vi "4155C Config Chart Colours.vi"(4 "Numeric":i32, 7 "XY Graph 2":refnum<vi>) -> ()   [LabVIEW 2019]
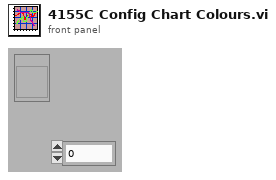
[diagram p1: front panel]
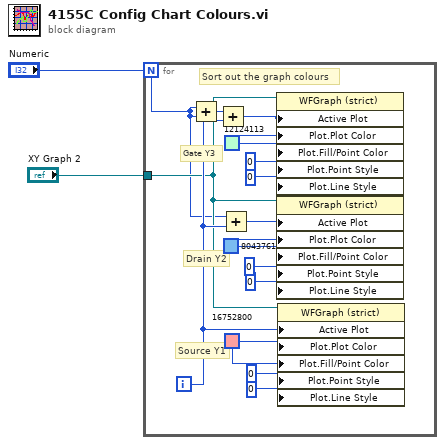
[diagram p0: block diagram]
diagram:
  n1 = for {
    N: "Numeric" -> [w3]
    tunnel: "XY Graph 2" -> [w6]
    i -> [w16]
    w15 = u32 16752800
    w14 = u32 8043761
    w13 = u32 12124113
    # "Sort out the graph colours"
    # "Source Y1"
    # "Drain Y2"
    # "Gate Y3"
    n2 = Add(x=w3, y=w3) -> (x+y=w17:i32)
    n3 = Add(x=w17, y=w16) -> (x+y=w5:i32)
    n4 = Add(x=w3, y=w16) -> (x+y=w4:i32)
    n5 = property on="Property Node" class="WFGraph (strict)"(reference=w6, "Active Plot"=w5, "Plot.Plot Color"=w13, "Plot.Fill/Point Color"=w13, "Plot.Point Style"=u8 0, "Plot.Line Style"=u8 0) -> ()  [unwired: 1 in, 2 out]
    n6 = property on="Property Node" class="WFGraph (strict)"(reference=w6, "Active Plot"=w4, "Plot.Plot Color"=w14, "Plot.Fill/Point Color"=w14, "Plot.Point Style"=u8 0, "Plot.Line Style"=u8 0) -> ()  [unwired: 1 in, 2 out]
    n7 = property on="Property Node" class="WFGraph (strict)"(reference=w6, "Active Plot"=w16, "Plot.Plot Color"=w15, "Plot.Fill/Point Color"=w15, "Plot.Point Style"=u8 0, "Plot.Line Style"=u8 0) -> ()  [unwired: 1 in, 2 out]
  }
